vi "FPGAmain_5761_v2.vi"() -> ()   [LabVIEW 2018]
uses:
  FPGA/DataMode.ctl
  FPGA/Input_5782/5782_Fast_PID_states.ctl
  <vilib>/Platform/TimedLoop/XDataNode/timing_clust.ctl
  <vilib>/Platform/TimedLoop/XDataNode/nitl_modes.ctl
  <vilib>/Platform/TimedLoop/XDataNode/wakeup.ctl
  <vilib>/rvi/Emulation/niFpgaGetClockAttributes.vi
  <vilib>/rvi/Emulation/niFpgaSctlEmulationGetInTimedLoop.vi
  <vilib>/rvi/Emulation/niFpgaEmulationReportErrorSimple.vi
  <vilib>/rvi/eio/common/nirviEmuTemplateMethod_errors.vi
  <vilib>/rvi/Emulation/niFpgaCriticalErrorInLSC.vi
  <vilib>/rvi/Emulation/niFpgaProcessEmulError.vi
  <vilib>/rvi/Emulation/niFpgaEmulationIsFPGAContextNoSignature.vi
  <vilib>/rvi/errors/niFpgaSetErrorForExecOnDevCompSimple.vi
  <vilib>/rvi/eio/common/nirviEmuReportErrorAndStop.vi
  <vilib>/rvi/DataTransferAndStorage/Container/Common/niFpgaContainerGetUniqueNameForEmu.vi
  <vilib>/rvi/FIFO/Fifo_Resource/nirvififoEmulationSetSize.vi
  <vilib>/rvi/FIFO/Fifo_Resource/nirviFifoEmulationQueueMgr.vi
  <instcachedir>/0/nirviFifoEmulationQueueMgr_E5CAEC123FF24DC58D834DCA3CDAA9B5.lvgen/nirviFifoEmulationQueueMgr_E5CAEC123FF24DC58D834DCA3CDAA9B5_016.vi
  <vilib>/rvi/FIFO/Fifo_Resource/nirvififoEmulationDetermineInputValidOut.vi
  <vilib>/rvi/FIFO/Fifo_Resource/nirvififoEmulationCreateLock.vi
  <vilib>/rvi/FIFO/Fifo_Resource/nirvififoEmulationObtainLock.vi
  <vilib>/rvi/FIFO/Fifo_Resource/nirvififoEmulationReleaseLock.vi
  <vilib>/rvi/occurrence/nirviWaitOnOccurrenceBase.vi
  <vilib>/rvi/errors/nirviReportUnexpectedCaseInternalError.vi
  <vilib>/rvi/errors/nirviReportUnexpectedCaseInternalError (U32).vi
  <vilib>/rvi/Memory/Memory_Emulation/niFpgaMemoryEmulationCacheClearOnFirstRun.vi
  <vilib>/rvi/Memory/Memory_Emulation/nirvimemoryEmulationManagerCache_MakeExclusive.vi
  <vilib>/rvi/Memory/Memory_Emulation/niFpgaMemoryEmulationValidateCache.vi
  <vilib>/rvi/Memory/Memory_Emulation/nirvimemoryEmulationManagerCache_InsertValue.vi
  <vilib>/Utility/error.llb/Clear Errors.vi
  <vilib>/rvi/Memory/Memory_Emulation/nirvimemoryEmulationManagerCache_ReleaseExclusive.vi
  <vilib>/rvi/Memory/Memory_Emulation/nirvimemoryEmulationManagerCache_GetValue.vi
  <vilib>/rvi/Memory/Memory_Emulation/nirvimemoryEmulationManagerCache_SetValue.vi
  <instcachedir>/0/nirviFifoEmulationQueueMgr_E5CAEC123FF24DC58D834DCA3CDAA9B5.lvgen/nirviFifoEmulationQueueMgr_E5CAEC123FF24DC58D834DCA3CDAA9B5_023.vi
  <vilib>/rvi/interface/RandomDataEmulation/niFpgaRandomDataHandleErrors.vi
  <vilib>/rvi/interface/RandomDataEmulation/nirviRandomDataMultiElementFPGAFIFO.vi
  <instcachedir>/0/nirviRandomDataMultiElementFPGAFIFO_6740B454F3C245F78F76ED91F73FD8DB.lvgen/nirviRandomDataMultiElementFPGAFIFO_6740B454F3C245F78F76ED91F73FD8DB_001.vi
  <vilib>/eio/EIONode/EIONode.xnode
  <vilib>/Platform/TimedLoop/XDataNode/XDataNode.xnode
  <vilib>/rvi/FXPMathLib/FxpInterpret/XNode/nifxpmath_Interpret.xnode
  <vilib>/rvi/DataTransferAndStorage/Container/XNode/niFpgaContainer.xnode
  <vilib>/rvi/FIFO/Fifo_Resource/nirvififoEmulationWrite.vi
  <vilib>/rvi/DataTransferAndStorage/Register/Emulation/niFpgaRegisterEmulation.vi
  <vilib>/rvi/FIFO/Fifo_Resource/nirvififoEmulationRead.vi
  <vilib>/rvi/interface/RandomDataEmulation/nirviRandomDataFpgaReadWriteTemplate.vi
  <vilib>/rvi/interface/RandomDataEmulation/nirviRandomDataFpgaMultiElementTemplate.vi
  <vilib>/Platform/TimedLoop/XDataNode/XDNodeRunTimeDep.lvlib
panel:
  in  "Sample Clock Commit":bool
  in  "Sample Clock Select":u8
  out "SPI Idle":bool
  out "Configuration Error":bool
  out "Synthesizer Locked":bool
  out "Configured?":bool
  in  "Full speed transfer":bool
  in  "Continuous":bool
  in  "Record length":u16=4000 caption="Samples Per Trigger" min=1 step=1
  in  "Trigger Acquisition":bool
  out "IO Module\\Trigger Input":bool
  in  "Acquisition running":bool
  in  "Simulated phase":fxp<+,64,64>[](array[numeric])=[0.0, 0.0]
  in  "Mode":T1
  in  "Phase input":fxp<+,64,64>[](array[numeric])=[0.0, 0.0, 0.0, 0.0, 0.0, 0.0, 0.0, 0.0, 0.0, 0.0, 0.0, 0.0, 0.0, 0.0, 0.0, 0.0]
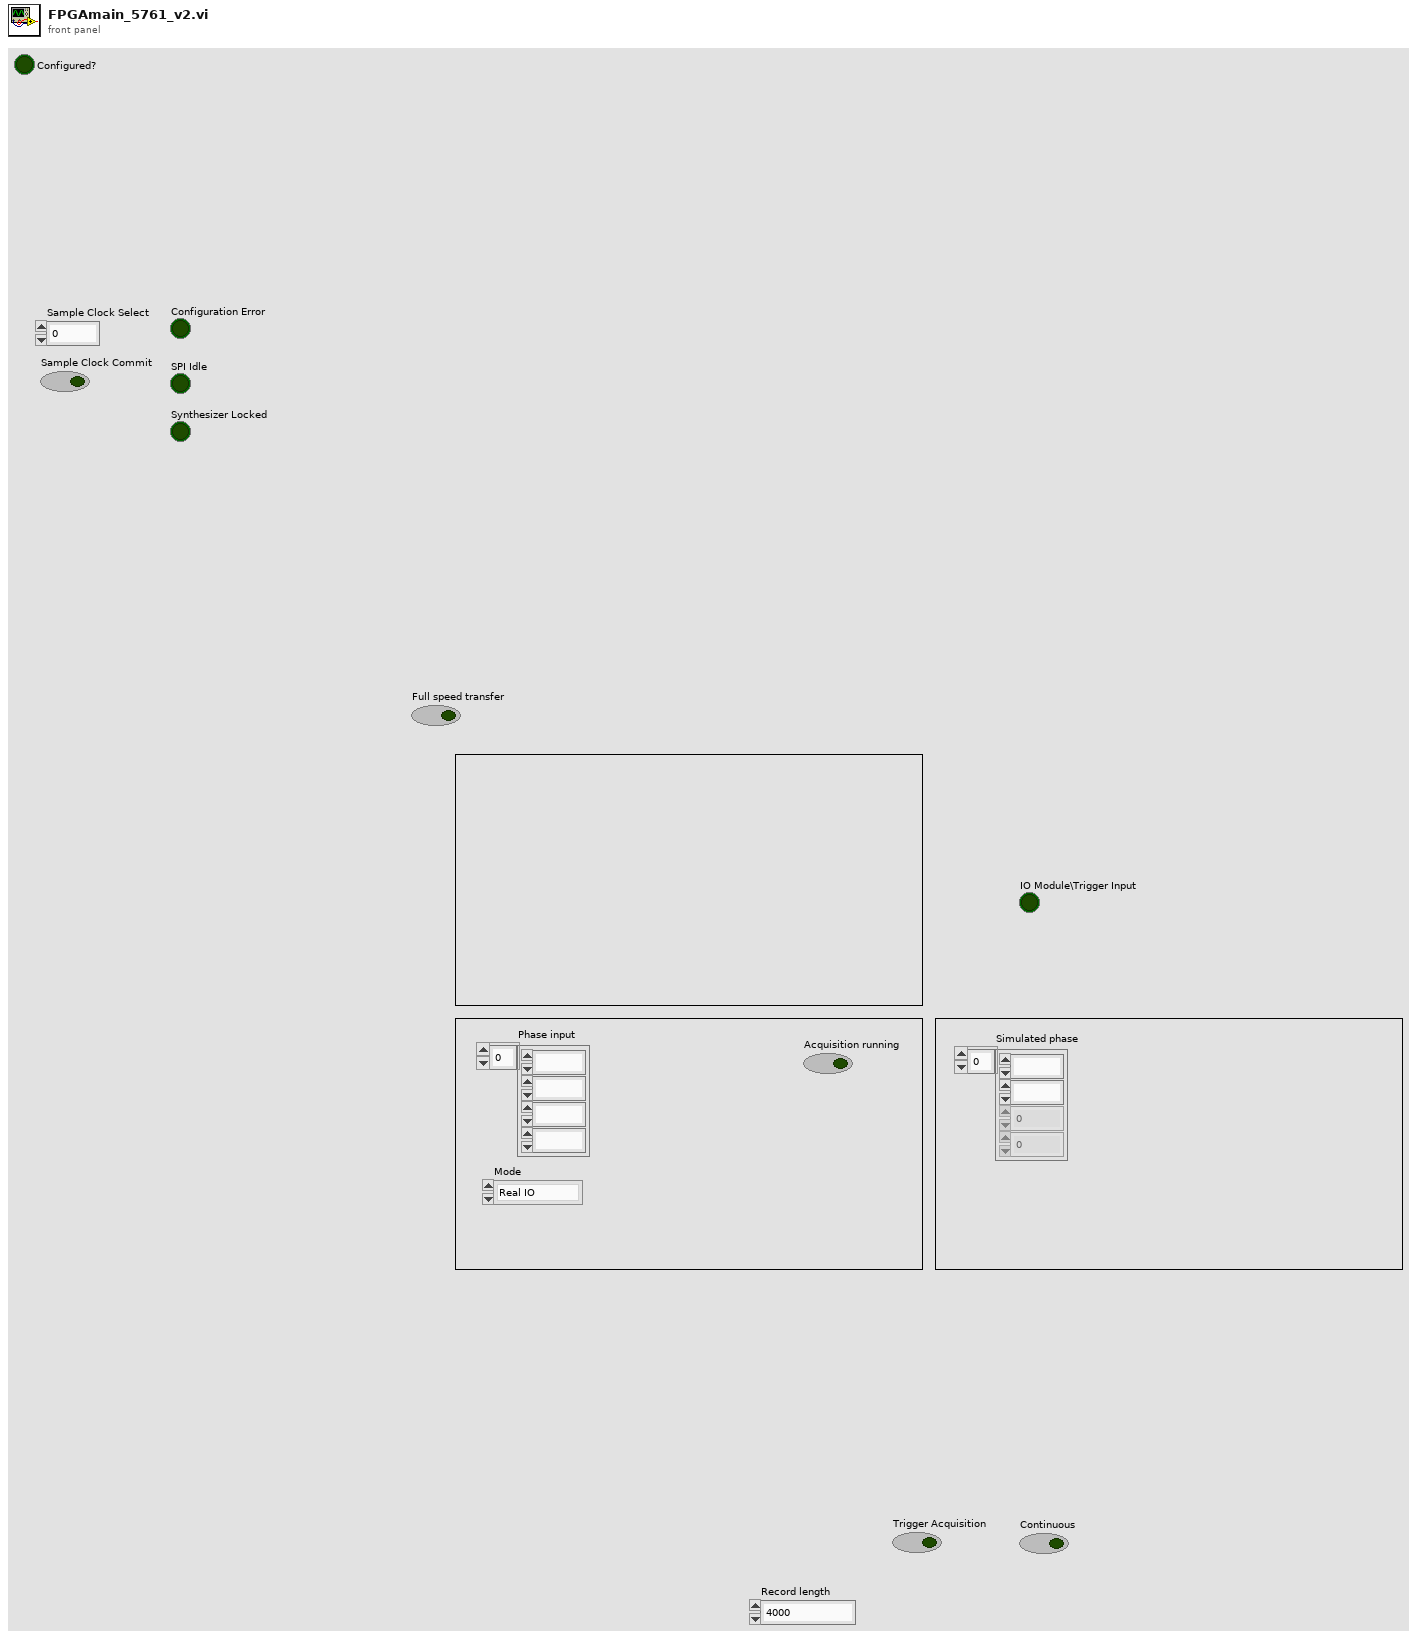
[diagram p1: front panel]
types:
  T1 = typedef "DataMode.ctl" = enum16{"Real IO", "Simulated"}
  T2 = typedef "5782_Fast_PID_states.ctl" = enum8{"Wait for trigger", "Acquisition", "Send record length", "Wait for output", "Quiet period"}
  T3 = typedef "XDNodeRunTimeDep.lvlib/timing_clust.ctl" = cluster{"Expected End [f-1]":u64, "Actual End [f-1]":u64, "Finished Late? [f-1]":bool, "Expected End [i-1]":u64, "Actual End [i-1]":u64, "Finished Late? [i-1]":bool, "Expected Start [i]":u64, "Actual Start [i]":u64, "Expected Start [f]":u64, "Actual Start [f]":u64, "Source Name":string, "Structure Name":string, "Period":i64, "Deadline":i64, "Offset":i64, "Start":i64, "Priority":i32, "Timeout":i32, "Mode":T4, "Wakeup Reason":T5, "Error":errorcluster, "Source Type":string, "Secondary Source Type":string, "Global End Time":u64, "Global Start Time":u64, "Frame Duration":u64, "Iteration Duration":u64, "Assigned CPU":i32, "I/O Scan Engine Mode":u32}
  T4 = typedef "XDNodeRunTimeDep.lvlib/nitl_modes.ctl" = enum32{"No Change", "Process missed periods, maintain original phase", "Discard missed periods, maintain original phase", "Process missed periods, ignore original phase", "Discard missed periods, ignore original phase"}
  T5 = typedef "XDNodeRunTimeDep.lvlib/wakeup.ctl" = enum32{"Normal", "Aborted", "Asynchronous wakeup", "Timing source error", "Timed loop error", "Timeout"}
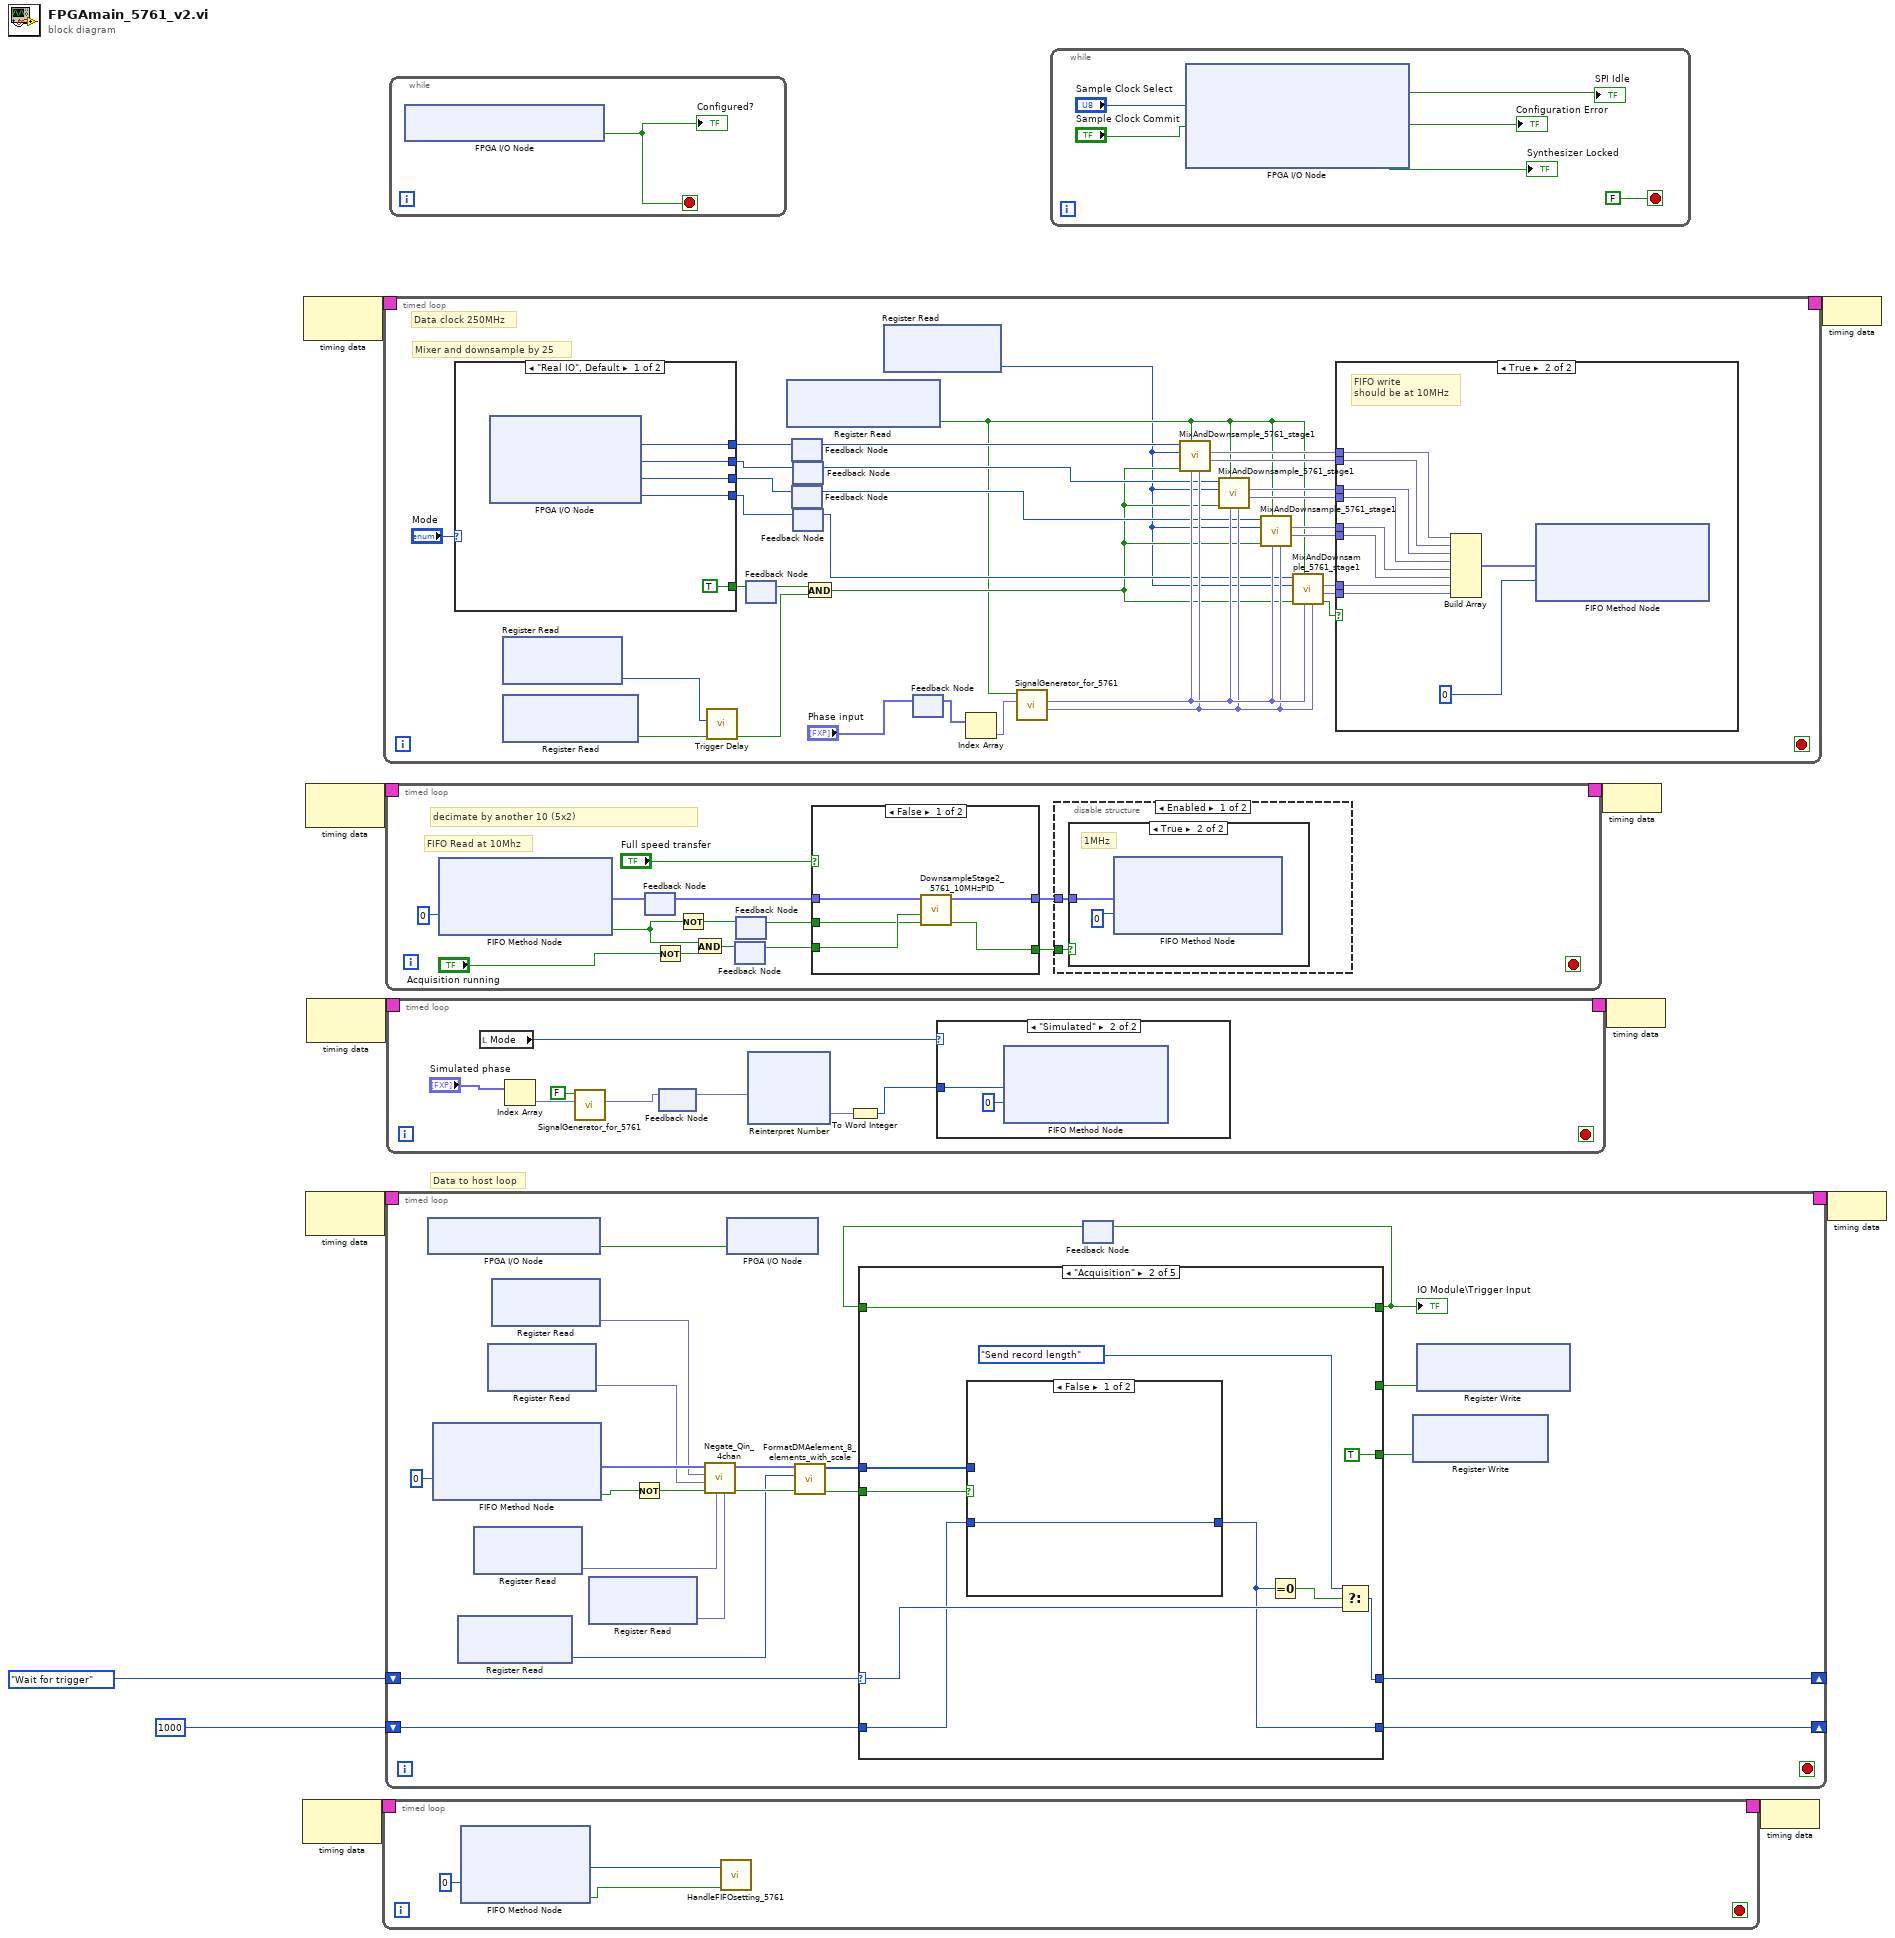
[diagram p0: block diagram]
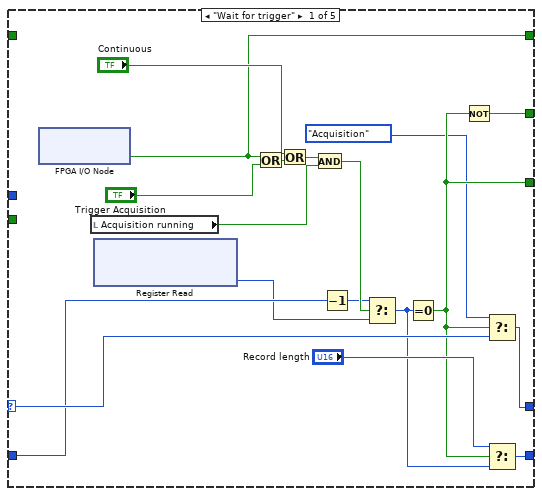
[diagram p2: hidden frame]
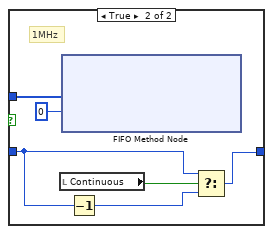
[diagram p3: hidden frame]
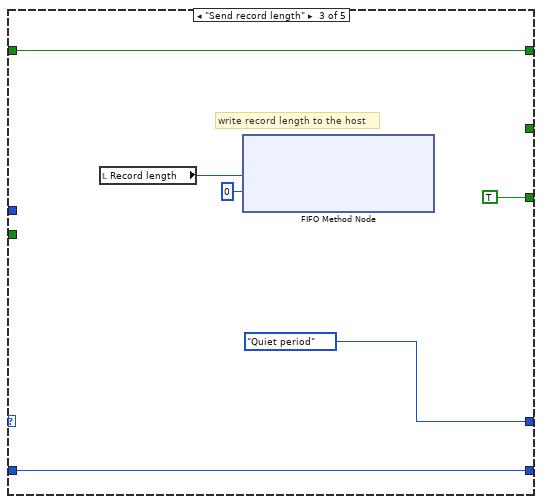
[diagram p4: hidden frame]
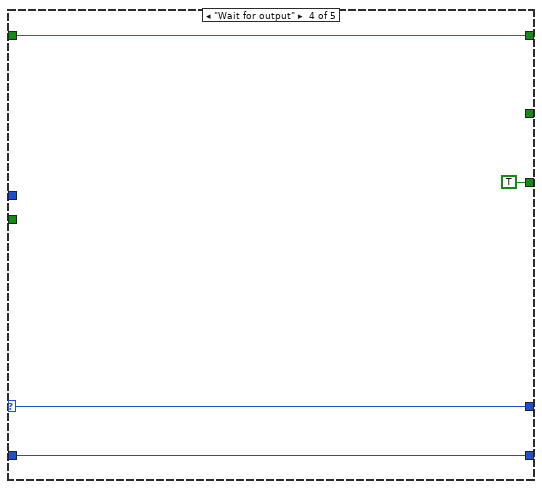
[diagram p5: hidden frame]
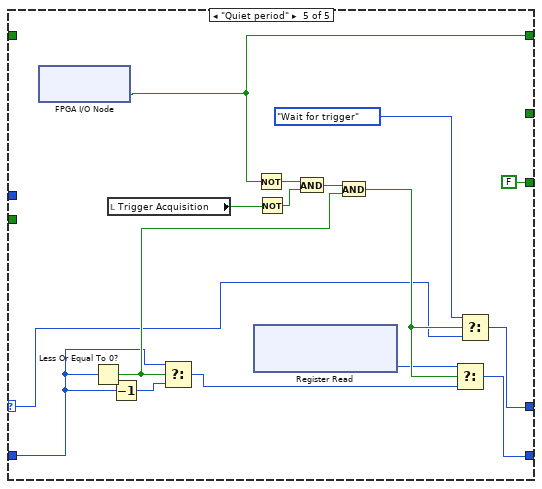
[diagram p6: hidden frame]
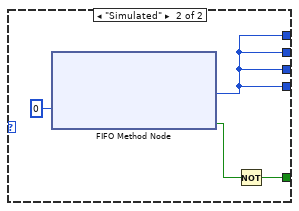
[diagram p11: hidden frame]
diagram:
  # "Data to host loop"
  n1 = node-c288() -> (w7:T3)  [unwired: 1 in]
  n2 = node-c288() -> (w10:T3)  [unwired: 1 in]
  n3 = node-c288() -> (w5:T3)  [unwired: 1 in]
  n4 = node-c288() -> (w3:T3)  [unwired: 1 in]
  n5 = node-c288() -> (w12:T3)  [unwired: 1 in]
  n6 = timed-loop {
    timing: w7 -> [_]
    timing-out: [_] -> w6
    stop <- _ stop-if-true
    n7 = xnode ("FIFO Method Node")("Timeout"=0) -> ("Element"=w14:u64, "Timed Out?"=w13:bool)  [unwired: 1 in, 1 out]
    n8 = call "HandleFIFOsetting_5761.vi"("timed out"=w13, "Value"=w14) -> ()  [unwired: 10 in]
  }
  n9 = timed-loop {
    timing: w10 -> [_]
    timing-out: [_] -> w9
    stop <- _ stop-if-true
    # "Mixer and downsample by 25"
    # "Data clock 250MHz"
    n10 = case shown="\"Real IO\", Default" "Mode" {
      tunnel: [TRUE w65] -> w47
      tunnel: [w62 w64] -> w44
      tunnel: [w61 w64] -> w43
      tunnel: [w60 w64] -> w42
      tunnel: [w59 w64] -> w41
      frame "Real IO", Default {
        n11 = xnode "FPGA I/O Node"() -> ("IO Module\\AI 0 Data"=w62:i16, "IO Module\\AI 1 Data"=w61:i16, "IO Module\\AI 2 Data"=w60:i16, "IO Module\\AI 3 Data"=w59:i16)  [unwired: 4 in, 4 out]
      }
      frame "Simulated" {
        n12 = xnode ("FIFO Method Node")("Timeout"=0) -> ("Element"=w64:i16, "Timed Out?"=w66:bool)  [unwired: 1 in, 1 out]
        n13 = Not(x=w66) -> (.not. x?=w65:bool)
      }
    }
    n14 = xnode ("Register Read")() -> ("Data"=w32:u32)  [unwired: 1 in, 1 out]
    n15 = xnode ("Register Read")() -> ("Data"=w31:bool)  [unwired: 1 in, 1 out]
    n16 = call "Trigger Delay.vi"("input valid"=w31, "Count to skip"=w32) -> ("output valid"=w30:bool)  [unwired: 9 in]
    n17 = feedback #1() -> (w46:bool)  [unwired: 1 in]
    n18 = feedback-in #1(w47) -> ()
    n19 = xnode ("Register Read")() -> ("Data"=w19:bool)  [unwired: 1 in, 1 out]
    n20 = feedback #2() -> (w40:i16)  [unwired: 1 in]
    n21 = feedback-in #2(w44) -> ()
    n22 = feedback #3() -> (w34:i16)  [unwired: 1 in]
    n23 = feedback-in #3(w42) -> ()
    n24 = feedback #4() -> (w35:i16)  [unwired: 1 in]
    n25 = feedback-in #4(w43) -> ()
    n26 = feedback #5() -> (w33:i16)  [unwired: 1 in]
    n27 = feedback-in #5(w41) -> ()
    n28 = And(x=w46, y=w30) -> (x .and. y?=w20:bool)
    n29 = xnode ("Register Read")() -> ("Data"=w18:u16)  [unwired: 1 in, 1 out]
    n30 = feedback #6() -> (w39:fxp<+,64,64>[])  [unwired: 1 in]
    n31 = feedback-in #6("Phase input") -> ()
    n32 = Index Array(array=w39) -> (element=w38:fxp<+,64,64>)  [unwired: 1 in]
    n33 = call "SignalGenerator_for_5761.vi"("phase"=w38, "Reset"=w19) -> ("Cos"=w36:fxp<+/-,16,0>, "Sin"=w37:fxp<+/-,16,0>)  [unwired: 7 in, 1 out]
    n34 = call "MixAndDownsample_5761_stage1.vi"("cosine"=w36, "sine"=w37, "reset"=w19, "Input Valid (T)"=w20, "factor"=w18, "Analog in"=w40) -> ("Q out"=w27:fxp<+/-,32,14>, "I out"=w28:fxp<+/-,32,14>)  [unwired: 3 in, 1 out]
    n35 = call "MixAndDownsample_5761_stage1.vi"("cosine"=w36, "sine"=w37, "reset"=w19, "Input Valid (T)"=w20, "factor"=w18, "Analog in"=w35) -> ("Q out"=w25:fxp<+/-,32,14>, "I out"=w26:fxp<+/-,32,14>)  [unwired: 3 in, 1 out]
    n36 = call "MixAndDownsample_5761_stage1.vi"("cosine"=w36, "sine"=w37, "reset"=w19, "Input Valid (T)"=w20, "factor"=w18, "Analog in"=w34) -> ("Q out"=w23:fxp<+/-,32,14>, "I out"=w24:fxp<+/-,32,14>)  [unwired: 3 in, 1 out]
    n37 = call "MixAndDownsample_5761_stage1.vi"("cosine"=w36, "sine"=w37, "reset"=w19, "Input Valid (T)"=w20, "factor"=w18, "Analog in"=w33) -> ("data valid"=w29:bool, "Q out"=w21:fxp<+/-,32,14>, "I out"=w22:fxp<+/-,32,14>)  [unwired: 3 in]
    n38 = case shown="True" w29 {
      tunnel: w28 -> [_ w56]
      tunnel: w27 -> [_ w55]
      tunnel: w26 -> [_ w54]
      tunnel: w25 -> [_ w53]
      tunnel: w24 -> [_ w52]
      tunnel: w23 -> [_ w51]
      tunnel: w22 -> [_ w50]
      tunnel: w21 -> [_ w49]
      frame False {
      }
      frame True {
        # "FIFO write\nshould be at 10MHz"
        n39 = Build Array(w56, w55, w54, w53, w52, w51, w50, w49) -> (w58:fxp<+/-,32,14>[])
        n40 = xnode ("FIFO Method Node")("Element"=w58, "Timeout"=0) -> ()  [unwired: 1 in, 2 out]
      }
    }
  }
  n41 = timed-loop {
    timing: w5 -> [_]
    timing-out: [_] -> w4
    stop <- _ stop-if-true
    # "FIFO Read at 10Mhz"
    # "decimate by another 10 (5x2)"
    n42 = xnode ("FIFO Method Node")("Timeout"=0) -> ("Element"=w78:fxp<+/-,32,14>[], "Timed Out?"=w79:bool)  [unwired: 1 in, 1 out]
    n43 = feedback #7() -> (w77:fxp<+/-,32,14>[])  [unwired: 1 in]
    n44 = feedback-in #7(w78) -> ()
    n45 = Not(x="Acquisition running") -> (.not. x?=w71:bool)
    n46 = Not(x=w79) -> (.not. x?=w73:bool)
    n47 = And(x=w79, y=w71) -> (x .and. y?=w75:bool)
    n48 = feedback #8() -> (w74:bool)  [unwired: 1 in]
    n49 = feedback-in #8(w75) -> ()
    n50 = feedback #9() -> (w72:bool)  [unwired: 1 in]
    n51 = feedback-in #9(w73) -> ()
    n52 = case shown="False" "Full speed transfer" {
      tunnel: [w91 w93] -> w81
      tunnel: [w90 w92] -> w80
      tunnel: w77 -> [w89 w93]
      tunnel: w74 -> [w88 _]
      tunnel: w72 -> [w87 w92]
      frame False {
        n53 = call "DownsampleStage2_5761_10MHzPID.vi"("valid in"=w87, "reset"=w88, "Data in"=w89) -> ("valid out"=w90:bool, "data out"=w91:fxp<+/-,32,14>[])  [unwired: 7 in]
      }
      frame True {
      }
    }
    n54 = disable-structure shown="Enabled" {
      disable-tunnel: w81 -> [w84 _]
      disable-tunnel: w80 -> [w83 _]
      frame Enabled {
        n55 = case shown="True" w83 {
          tunnel: w84 -> [_ w85]
          frame False {
          }
          frame True {
            # "1MHz"
            n56 = xnode ("FIFO Method Node")("Element"=w85, "Timeout"=0) -> ()  [unwired: 1 in, 2 out]
          }
        }
      }
      frame Disabled {
      }
    }
  }
  n57 = timed-loop {
    timing: w3 -> [_]
    timing-out: [_] -> w2
    shift-right: [w115] -> _
    shift-left: 5782_Fast_PID_states."Wait for trigger" ("5782 states") -> [w117]
    shift-right: [w114] -> _
    shift-left: u16 1000 ("trigger samples") -> [w116]
    stop <- _ stop-if-true
    n58 = xnode "FPGA I/O Node"() -> ("IO Module\\Trigger Input"=w97:bool)  [unwired: 1 in, 1 out]
    n59 = xnode ("FIFO Method Node")("Timeout"=0) -> ("Element"=w107:fxp<+/-,32,14>[], "Timed Out?"=w112:bool)  [unwired: 1 in, 1 out]
    n60 = xnode ("Register Read")() -> ("Data"=w96:u16)  [unwired: 1 in, 1 out]
    n61 = xnode ("Register Read")() -> ("Data"=w101:fxp<+/-,32,14>)  [unwired: 1 in, 1 out]
    n62 = xnode ("Register Read")() -> ("Data"=w102:fxp<+/-,32,14>)  [unwired: 1 in, 1 out]
    n63 = xnode ("Register Read")() -> ("Data"=w103:fxp<+/-,32,14>)  [unwired: 1 in, 1 out]
    n64 = xnode ("Register Read")() -> ("Data"=w100:fxp<+/-,32,14>)  [unwired: 1 in, 1 out]
    n65 = Not(x=w112) -> (.not. x?=w105:bool)
    n66 = call "Negate_Qin_4chan.vi"("DC offset chan 3"=w100, "DC offset chan 2"=w101, "valid in"=w105, "DC offset chan 1"=w102, "DC offset chan 0"=w103, "Data in"=w107) -> ("valid out"=w104:bool, "Data out"=w106:fxp<+/-,32,14>[])  [unwired: 4 in]
    n67 = xnode "FPGA I/O Node"("PXI_Trig0"=w97) -> ()  [unwired: 1 in, 1 out]
    n68 = call "FormatDMAelement_8_elements_with_scale.vi"("valid in"=w104, "factor"=w96, "Data in"=w106) -> ("valid out"=w110:bool, "Values"=w109:u64[])  [unwired: 7 in]
    n69 = feedback #10() -> (w98:bool)  [unwired: 1 in]
    n70 = case shown="\"Acquisition\"" w117 {
      selector: w117 -> [w135 w145 _ w160 w165]
      tunnel: w116 -> [w126 w142 w153 w159 w166]
      tunnel: [w134 w144 5782_Fast_PID_states."Quiet period" ("5782 states") w160 w177] -> w115
      tunnel: [w133 w139 w153 w159 w178] -> w114
      tunnel: w109 -> [_ w140 _ _ _]
      tunnel: w110 -> [_ w141 _ _ _]
      tunnel: [w121 TRUE TRUE ("5782 triggered") TRUE ("5782 triggered") FALSE ("5782 triggered")] -> w111
      tunnel: [w118 w138 w155 w161 w163] -> w99
      tunnel: w98 -> [_ w138 w155 w161 _]
      tunnel: [w120 _ _ _ _] -> w108
      frame "Wait for trigger" {
        n71 = xnode "FPGA I/O Node"() -> ("PXI_Trig0"=w118:bool)  [unwired: 1 in, 1 out]
        n72 = local read "Acquisition running"() -> (w129:bool)
        n73 = xnode ("Register Read")() -> ("Data"=w122:u16)  [unwired: 1 in, 1 out]
        n74 = Or(x=w118, y="Trigger Acquisition") -> (x .or. y?=w125:bool)
        n75 = Or(x="Continuous", y=w125) -> (x .or. y?=w123:bool)
        n76 = And(x=w123, y=w129) -> (x .and. y?=w130:bool)
        n77 = Decrement(x=w126) -> (x-1=w127:u16)
        n78 = Select(t=w127, s=w130, f=w122) -> (s? t:f=w128:u16)
        n79 = Equal To 0?(x=w128) -> (x = 0?=w121:bool)
        n80 = Not(x=w121) -> (.not. x?=w120:bool)
        n81 = Select(t=5782_Fast_PID_states."Acquisition" ("5782 states"), s=w121, f=w135) -> (s? t:f=w134:T2)
        n82 = Select(t="Record length", s=w121, f=w128) -> (s? t:f=w133:u16)
      }
      frame "Acquisition" {
        n83 = case shown="False" w141 {
          tunnel: w140 -> [_ w152]
          tunnel: [w146 w149] -> w139
          tunnel: w142 -> [w146 w147]
          frame False {
          }
          frame True {
            # "1MHz"
            n84 = local read "Continuous"() -> (w150:bool)
            n85 = xnode ("FIFO Method Node")("Element"=w152, "Timeout"=0) -> ()  [unwired: 1 in, 2 out]
            n86 = Decrement(x=w147) -> (x-1=w148:u16)
            n87 = Select(t=w147, s=w150, f=w148) -> (s? t:f=w149:u16)
          }
        }
        n88 = Equal To 0?(x=w139) -> (x = 0?=w143:bool)
        n89 = Select(t=5782_Fast_PID_states."Send record length" ("5782 states"), s=w143, f=w145) -> (s? t:f=w144:T2)
      }
      frame "Send record length" {
        # "write record length to the host"
        n90 = local read "Record length"() -> (w157:u16)
        n91 = xnode ("FIFO Method Node")("Element"=w157, "Timeout"=0) -> ()  [unwired: 1 in, 2 out]
      }
      frame "Wait for output" {
      }
      frame "Quiet period" {
        n92 = xnode "FPGA I/O Node"() -> ("PXI_Trig0"=w163:bool)  [unwired: 1 in, 1 out]
        n93 = Less Or Equal To 0?(x=w166) -> (x <= 0?=w169:bool)
        n94 = local read "Trigger Acquisition"() -> (w175:bool)
        n95 = Decrement(x=w166) -> (x-1=w170:u16)
        n96 = Select(t=w166, s=w169, f=w170) -> (s? t:f=w168:u16)
        n97 = xnode ("Register Read")() -> ("Data"=w167:u16)  [unwired: 1 in, 1 out]
        n98 = Not(x=w163) -> (.not. x?=w174:bool)
        n99 = Not(x=w175) -> (.not. x?=w173:bool)
        n100 = And(x=w174, y=w173) -> (x .and. y?=w172:bool)
        n101 = And(x=w172, y=w169) -> (x .and. y?=w176:bool)
        n102 = Select(t=w167, s=w176, f=w168) -> (s? t:f=w178:u16)
        n103 = Select(t=5782_Fast_PID_states."Wait for trigger" ("5782 states"), s=w176, f=w165) -> (s? t:f=w177:T2)
      }
    }
    "IO Module\\Trigger Input" <- w99
    n104 = feedback-in #10(w99) -> ()
    n105 = xnode ("Register Write")("Data"=w111) -> ()  [unwired: 1 in, 1 out]
    n106 = xnode ("Register Write")("Data"=w108) -> ()  [unwired: 1 in, 1 out]
  }
  n107 = timed-loop {
    timing: w12 -> [_]
    timing-out: [_] -> w11
    stop <- _ stop-if-true
    n108 = local read "Mode"() -> (w188:T1)
    n109 = Index Array(array="Simulated phase") -> (element=w187:fxp<+,64,64>)  [unwired: 1 in]
    n110 = call "SignalGenerator_for_5761.vi"("phase"=w187, "Reset"=FALSE) -> ("Sin"=w182:fxp<+/-,16,0>)  [unwired: 7 in, 2 out]
    n111 = feedback #11() -> (w183:fxp<+/-,16,0>)  [unwired: 1 in]
    n112 = feedback-in #11(w182) -> ()
    n113 = xnode "Reinterpret Number"("x"=w183) -> ("y"=w184:fxp<+/-,16,13>)
    n114 = To Word Integer(number=w184) -> (16bit integer=w181:i16)
    n115 = case shown="\"Simulated\"" w188 {
      tunnel: w181 -> [_ w189]
      frame "Real IO", Default {
      }
      frame "Simulated" {
        n116 = xnode ("FIFO Method Node")("Element"=w189, "Timeout"=0) -> ()  [unwired: 1 in, 2 out]
      }
    }
  }
  n117 = while {
    stop <- w193 stop-if-true
    n118 = xnode "FPGA I/O Node"() -> ("IO Module\\Initialization Done"=w193:bool)  [unwired: 1 in, 1 out]
    "Configured?" <- w193
  }
  n119 = while {
    stop <- FALSE stop-if-true
    n120 = xnode "FPGA I/O Node"("IO Module\\Sample Clock Select"="Sample Clock Select", "IO Module\\Sample Clock Commit"="Sample Clock Commit") -> ("IO Module\\SPI Idle"=→"SPI Idle":bool, "IO Module\\Configuration Error"=→"Configuration Error":bool, "IO Module\\Synthesizer Locked"=→"Synthesizer Locked":bool)  [unwired: 5 in, 5 out]
  }
  n121 = node-c288(w4) -> ()
  n122 = node-c288(w11) -> ()
  n123 = node-c288(w6) -> ()
  n124 = node-c288(w9) -> ()
  n125 = node-c288(w2) -> ()
